vi "setMode.vi"(8 "error in (no error)":errorcluster, 10 "Measurement Function (0: Current)":i32(ring) items=["Current", "Charge", "Voltage", "Resistance"], 11 "Electrometer in":refnum<class "Electrometer.lvclass">) -> (0 "error out":errorcluster, 3 "Electrometer out":refnum<class "Electrometer.lvclass">)   [LabVIEW 2016, in "Electrometer.lvclass"]
uses:
  Electrometer.lvclass
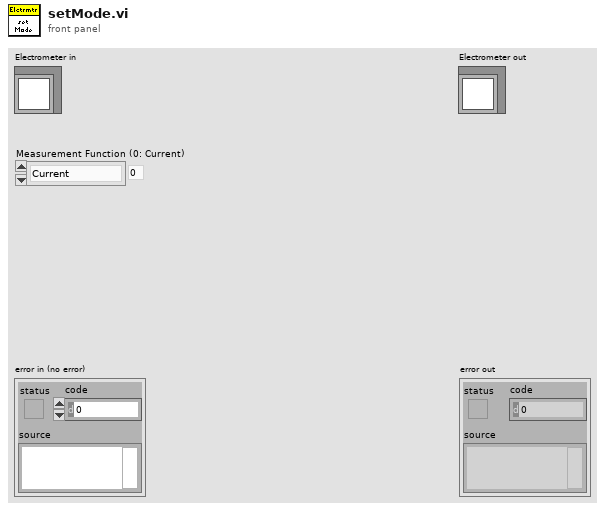
[diagram p1: front panel]
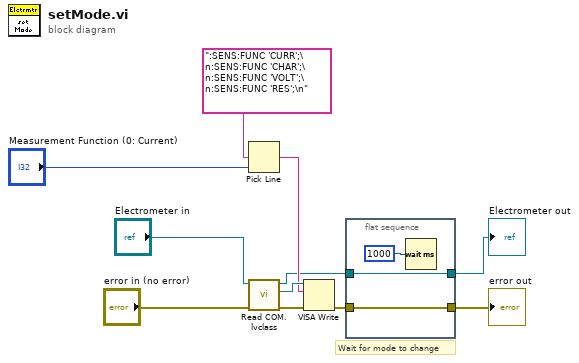
[diagram p0: block diagram]
diagram:
  # "Wait for mode to change"
  n1 = Pick Line(multi-line string=":SENS:FUNC 'CURR';\n:SENS:FUNC 'CHAR';\n:SENS:FUNC 'VOLT';\n:SENS:FUNC 'RES';\n", line index="Measurement Function (0: Current)") -> (output string=w8:string)  [unwired: 1 in]
  n2 = call "Read COM.lvclass.vi"("error in (no error)"="error in (no error)", "Electrometer in"="Electrometer in") -> ("error out"=w6:errorcluster, "VISA"=w9:refnum<visa-resource-name>, "Electrometer out"=w4:refnum<class "Electrometer.lvclass">)  [unwired: 7 in]
  n3 = VISA Write(VISA resource name=w9, write buffer=w8, error in (no error)=w6) -> (error out=w5:errorcluster)  [unwired: 2 out]
  n4 = flat-sequence {
    tunnel: w4 -> [w14]
    tunnel: [w14] -> w3
    tunnel: w5 -> [w13]
    tunnel: [w13] -> w2
    frame #0 {
      n5 = Wait (ms)(milliseconds to wait=u32 1000) -> ()  [unwired: 1 out]
    }
  }
  "error out" <- w2
  "Electrometer out" <- w3
